vi "Read E and F Params.vi"(8 "error in (no error)":errorcluster, 11 "BME_DG_G08_Chnl in":refnum<class "BME_DG_G05P2_Chnl.lvclass">) -> (0 "error out":errorcluster, 2 "Disconnect (E,F)":bool, 3 "BME_DG_G08_Chnl out":refnum<class "BME_DG_G05P2_Chnl.lvclass">)   [LabVIEW 2009]
uses:
  BME_DG_G05P2_Chnl.lvclass
panel:
  out "Input Positive (E,F)":bool
  out "OntoMsBus (E,F)":bool
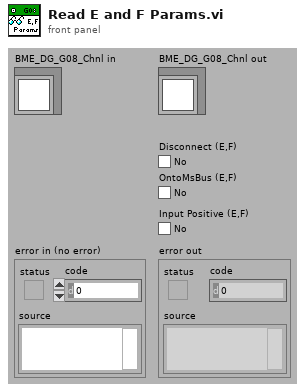
[diagram p1: front panel]
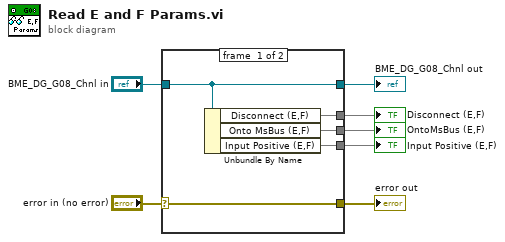
[diagram p0: block diagram]
diagram:
  n1 = case shown="No Error" "error in (no error)" {
    selector: "error in (no error)" -> [w12 w13]
    tunnel: [w12 w13] -> w6
    tunnel: [w11 w14] -> w4
    tunnel: "BME_DG_G08_Chnl in" -> [w11 w14]
    tunnel: [w10 _] -> w3
    tunnel: [w9 _] -> w2
    tunnel: [w8 _] -> w1
    frame #0 {
      n2 = Unbundle By Name(w11) -> ("Disconnect (E,F)"=w10, "Onto MsBus (E,F)"=w9, "Input Positive (E,F)"=w8)
    }
    frame #1 {
    }
  }
  "error out" <- w6
  "BME_DG_G08_Chnl out" <- w4
  "Disconnect (E,F)" <- w3
  "OntoMsBus (E,F)" <- w2
  "Input Positive (E,F)" <- w1
